vi "LVCAM Propagate Error.vi"(10 "Error":errorcluster, 11 "Self Actor in":refnum<class "Self Actor.lvclass">) -> (3 "Self Actor out":refnum<class "Self Actor.lvclass">)   [LabVIEW 2021, in "LVCAM.lvlib" / "Self Actor.lvclass"]
uses:
  Self Actor.lvclass
  C:/PPLs/LabVIEW-Composed-Actor-Model-LVCAM/LabVIEW-Composed-Actor-Model-LVCAM/AAM/LVCAM/LVCAM/LVCAM.lvclass
  Self Actor.lvclass/Self Actor.ctl
  Msgs/LVCAM Destroy Self/LVCAM Destroy Self Msg/LVCAM Destroy Self Msg.lvclass
  C:/PPLs/LabVIEW-Composed-Actor-Model-LVCAM/LabVIEW-Composed-Actor-Model-LVCAM/AAM/LVCAM/Msg/Msg.lvclass
  Self Msg Send.vi
  LVCAM/LVCAM.lvclass
  C:/PPLs/LabVIEW-Composed-Actor-Model-LVCAM/LabVIEW-Composed-Actor-Model-LVCAM/AAM/Msgs/LVCAM Create Nest/LVCAM Create Nest/LVCAM Create Nest.lvclass
  C:/PPLs/LabVIEW-Composed-Actor-Model-LVCAM/LabVIEW-Composed-Actor-Model-LVCAM/AAM/Msgs/LVCAM Destroy Self/LVCAM Destroy Self/LVCAM Destroy Self.lvclass
  C:/PPLs/LabVIEW-Composed-Actor-Model-LVCAM/LabVIEW-Composed-Actor-Model-LVCAM/AAM/Msgs/LVCAM Nest Destroyed/LVCAM Nest Destroyed/LVCAM Nest Destroyed.lvclass
  C:/PPLs/LabVIEW-Composed-Actor-Model-LVCAM/LabVIEW-Composed-Actor-Model-LVCAM/AAM/LVCAM/LVCAM Msg Drop/LVCAM Msg Drop.lvclass
  C:/PPLs/LabVIEW-Composed-Actor-Model-LVCAM/LabVIEW-Composed-Actor-Model-LVCAM/AAM/LVCAM/LVCAM Msg Receive/LVCAM Msg Receive.lvclass
  C:/PPLs/LabVIEW-Composed-Actor-Model-LVCAM/LabVIEW-Composed-Actor-Model-LVCAM/AAM/LVCAM/LVCAM Propagate Error/LVCAM Propagate Error.lvclass
  C:/PPLs/LabVIEW-Composed-Actor-Model-LVCAM/LabVIEW-Composed-Actor-Model-LVCAM/AAM/LVCAM/LVCAM Write LVCAM/LVCAM Write LVCAM.lvclass
  C:/PPLs/LabVIEW-Composed-Actor-Model-LVCAM/LabVIEW-Composed-Actor-Model-LVCAM/AAM/LVCAM/Self Actor/Self Actor.lvclass
  C:/PPLs/LabVIEW-Composed-Actor-Model-LVCAM/LabVIEW-Composed-Actor-Model-LVCAM/AAM/Msgs/LVCAM Destroy Self/LVCAM Destroy Self Msg/LVCAM Destroy Self Msg.lvclass
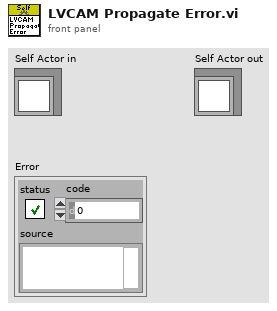
[diagram p1: front panel]
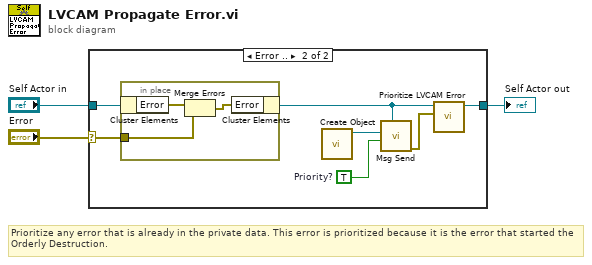
[diagram p0: block diagram]
diagram:
  # "Prioritize any error that is already in the private data. This error is prioritized because it is the error that started the Orderly Destruction."
  n1 = case shown="Error .." "Error" {
    selector: "Error" -> [_ w5]
    tunnel: "Self Actor in" -> [w4 w7]
    tunnel: [w4 w11] -> w2
    frame No Error {
    }
    frame Error {
      w8 = TRUE  # Priority?
      n2 = in-place {
        in-place-border: w5 -> [w14]
        n3 = in-place-cluster #1(w7) -> ("Error"=w12:errorcluster)
        n4 = Merge Errors(w12, w14) -> (w13:errorcluster)
        n5 = in-place-cluster #1("Error"=w13) -> (w6:refnum<class "Self Actor.lvclass">)
      }
      n6 = call "Create Object.vi"() -> ("LVCAM Destroy Self Msg out"=w9:refnum<class "LVCAM Destroy Self Msg.lvclass">)  [unwired: 11 in]
      n7 = call-poly "Msg Send.vi"("LVCAM"=w6, "Priority?"=w8, "Msg"=w9) -> ("error out"=w10:errorcluster)  [unwired: 8 in]
      n8 = call "Prioritize LVCAM Error.vi"("Error from LVCAM"=w10, "Self Actor in"=w6) -> ("Self Actor out"=w11:refnum<class "Self Actor.lvclass">)  [unwired: 9 in]
    }
  }
  "Self Actor out" <- w2
